vi "close.vi"(8 "error in (no error)":errorcluster caption="错误输入（无错误）", 11 "TCP_client 输入":refnum<class "TCP_client.lvclass">) -> (0 "error out":errorcluster caption="错误输出", 3 "TCP_client 输出":refnum<class "TCP_client.lvclass">)   [LabVIEW 2016, in "update.lvlib" / "TCP_client.lvclass"]
uses:
  TCP_client.lvclass
  TCP_client.lvclass/TCP_client.ctl
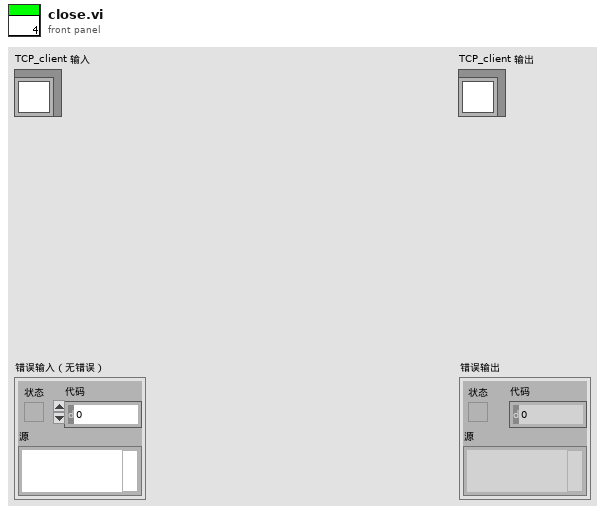
[diagram p1: front panel]
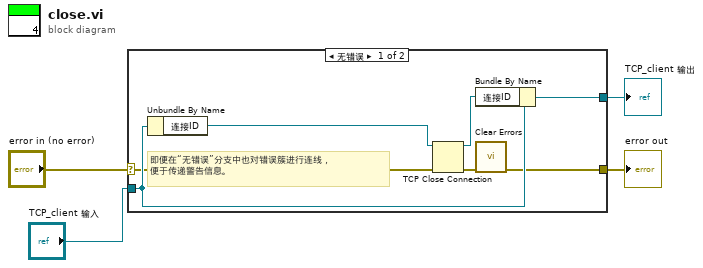
[diagram p0: block diagram]
diagram:
  n1 = case shown="无错误" "error in (no error)" {
    selector: "error in (no error)" -> [w9 w13]
    tunnel: [w7 w13] -> w3
    tunnel: [w5 w12] -> w1
    tunnel: "TCP_client 输入" -> [w11 w12]
    frame No Error {
      # "即便在“无错误”分支中也对错误簇进行连线，\n便于传递警告信息。"
      n2 = Unbundle By Name(w11) -> ("连接ID"=w10:refnum<k5>)
      n3 = TCP Close Connection(connection ID=w10, error in (no error)=w9) -> (connection ID out=w6:refnum<k5>, error out=w8:errorcluster)  [unwired: 1 in]
      n4 = Bundle By Name(cluster=w11, "连接ID"=w6) -> (w5:refnum<class "TCP_client.lvclass">)
      n5 = call <vilib>:"Clear Errors.vi"("error in (no error)"=w8) -> ("error out"=w7:errorcluster)  [unwired: 5 in, 1 out]
    }
    frame Error {
    }
  }
  "error out" <- w3
  "TCP_client 输出" <- w1
